vi "GV-SetGraphData.vi"(8 "error in (no error)":errorcluster, 9 "GviewerUpdate":T1, 11 "Gviewer in":refnum<class "Gviewer.lvclass">) -> (0 "error out":errorcluster, 3 "Gviewer out":refnum<class "Gviewer.lvclass">)   [LabVIEW 2020, in "Gviewer.lvclass"]
doc: "Andre Koelewijn, 17 jan 2021\n\nWrite Graph data"
uses:
  Gviewer.lvclass
  FAMM/controls/FAMM_reply_datagram.ctl
  controls/Typedef_Live.ctl
  FAMM/controls/FAMM_reply_PAQdata.ctl
  FAMM/controls/FAMM_reply_WAQdata.ctl
  FAMM/controls/FAMM_reply_EAQdata.ctl
  Gviewer.lvclass/Gviewer.ctl
  FAMM/FAMM.lvclass
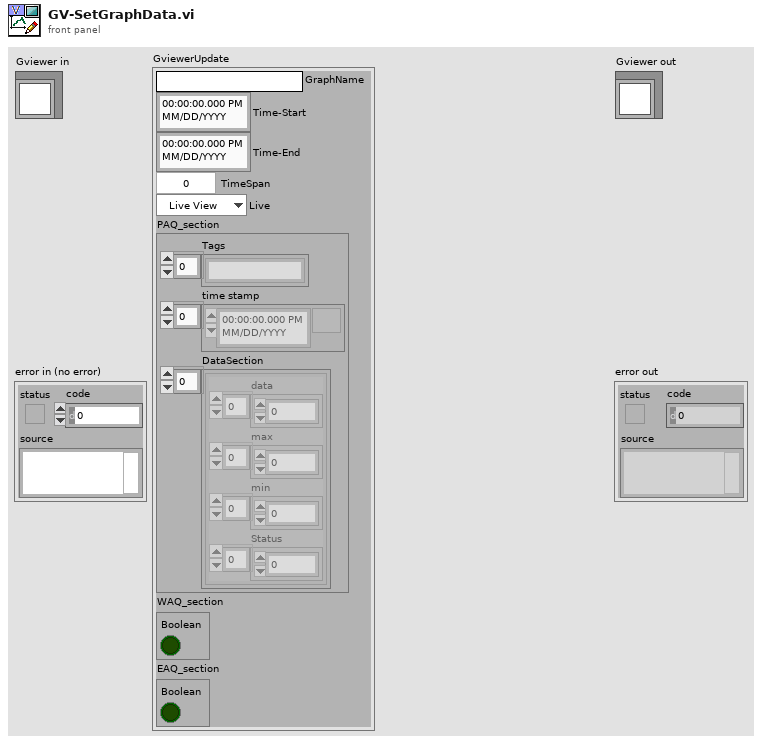
[diagram p1: front panel]
types:
  T1 = typedef "FAMM.lvclass/FAMM_reply_datagram.ctl" = cluster{"GraphName":string, "Time-Start":timestamp, "Time-End":timestamp, "TimeSpan":dbl, "Live":T2, "PAQ_section":T3, "WAQ_section":T4, "EAQ_section":T5}
  T2 = typedef "Gviewer.lvclass/Typedef_Live.ctl" = enum16{"Live View", "Freeze"}
  T3 = typedef "FAMM.lvclass/FAMM_reply_PAQdata.ctl" = cluster{"Tags":string[], "time stamp":timestamp[], "DataSection":cluster{"data":dbl[], "max":dbl[], "min":dbl[], "Status":u32[]}[]}
  T4 = typedef "FAMM.lvclass/FAMM_reply_WAQdata.ctl" = cluster{"Boolean":bool}
  T5 = typedef "FAMM.lvclass/FAMM_reply_EAQdata.ctl" = cluster{"Boolean":bool}
  T6 = cluster{"data":dbl[], "max":dbl[], "min":dbl[], "Status":u32[]}[]
  T7 = typedef "Gviewer.lvclass/Typedef_SelProperties.ctl" = cluster{"Color":u32, "LineType":T8, "max":dbl, "min":dbl}
  T8 = typedef "Gviewer.lvclass/Typedef_LineType.ctl" = enum16{"num_bare", "num_MinMax_Area", "num_MinMax_Lines", "num_MinMax_Forfor", "num_Max_Area", "num_Max_Line", "num_Max_Forfor", "num_Min_Area", "num_Min_Line", "num_Min_Fosfor", "Boolean_Line_01", "Boolean_Area_01", "Boolean_Fosfor_01", "Boolean_Line_TF", "Boolean_Area_TF", "Boolean_Fosfor_TF", "Boolean_OnOff_Line", "Boolean_OnOff_Area", "Boolean_OnOff_Fosfor", "Boolean_spare", "StringEvent_Line", "StringEvent_TimeLine"}
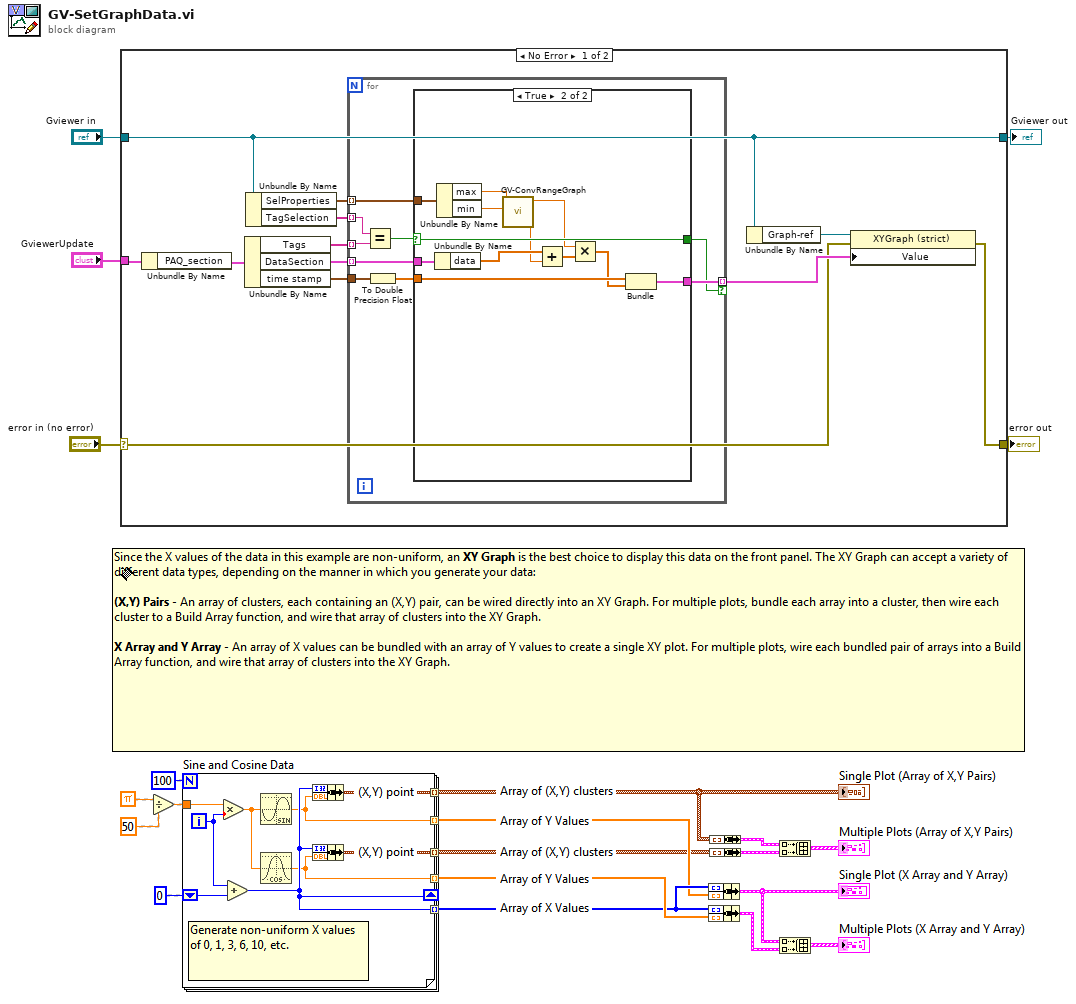
[diagram p0: block diagram]
diagram:
  n1 = case shown="No Error" "error in (no error)" {
    selector: "error in (no error)" -> [w8 w41]
    tunnel: [w7 w41] -> w4
    tunnel: [w11 w40] -> w2
    tunnel: "Gviewer in" -> [w11 w40]
    tunnel: "GviewerUpdate" -> [w17 _]
    frame No Error {
      n2 = Unbundle By Name(w17) -> ("PAQ_section"=w16:T3)
      n3 = Unbundle By Name(w16) -> ("Tags"=w15:string[], "DataSection"=w14:T6, "time stamp"=w13:timestamp[])
      n4 = Unbundle By Name(w11) -> ("SelProperties"=w6:T7[], "TagSelection"=w12:string[])
      n5 = for {
        tunnel: w15 -> [w26] mode=indexing
        tunnel: w14 -> [w23] mode=indexing
        tunnel: w13 -> [w22]
        tunnel: w12 -> [w25] mode=indexing
        tunnel: [w21] -> w9 mode=indexing if=w18
        tunnel: w6 -> [w19] mode=indexing
        n6 = Equal?(x=w25, y=w26) -> (x = y?=w24:bool)
        n7 = To Double Precision Float(number=w22) -> (double precision float=w20:dbl[])
        n8 = case shown="True" w24 {
          selector: w24 -> [w27 w36]
          tunnel: w23 -> [_ w38]
          tunnel: w20 -> [_ w39]
          tunnel: [_ w37] -> w21
          tunnel: [w27 w36] -> w18
          tunnel: w19 -> [_ w35]
          frame False {
          }
          frame True {
            n9 = Unbundle By Name(w38) -> ("data"=w32:dbl[])
            n10 = Unbundle By Name(w35) -> ("max"=w34:dbl, "min"=w33:dbl)
            n11 = call "GV-ConvRangeGraph.vi"("RangeL"=w33, "RangeH"=w34) -> ("Offset"=w28:dbl, "Gain"=w29:dbl)  [unwired: 8 in]
            n12 = Add(x=w32, y=w28) -> (x+y=w31:dbl[])
            n13 = Multiply(x=w29, y=w31) -> (x*y=w30:dbl[])
            n14 = Bundle(w39, w30) -> (w37:cluster{dbl[], dbl[]})  [unwired: 1 in]
          }
        }
      }
      n15 = Unbundle By Name(w11) -> ("Graph-ref"=w10:refnum<vi>)
      n16 = property class="XYGraph (strict)"(reference=w10, error in=w8, "Value"=w9) -> (error out=w7:errorcluster)  [unwired: 1 out]
    }
    frame Error {
    }
  }
  "error out" <- w4
  "Gviewer out" <- w2
